vi "WRITE Config to XML file.vi"(8 "error in (no error)":errorcluster, 10 "Path":path) -> (0 "error out":errorcluster)   [LabVIEW 2015, in "Tool Module.lvlib"]
uses:
  Tool Module.lvlib
  <vilib>/Utility/xml.llb/Write to XML File(array).vi
  Tool Config/Tool Cfg.lvlib
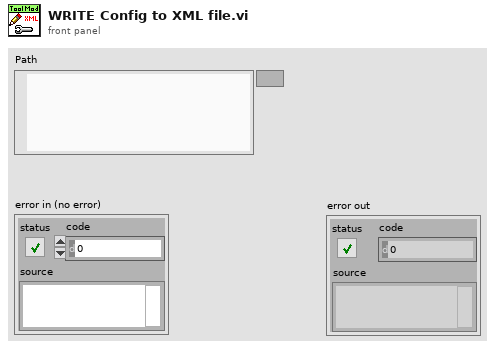
[diagram p1: front panel]
types:
  T1 = typedef "Tool Cfg.lvlib/_Configuration Cluster_v3--typedef.ctl" = cluster{"Tool Type":u16, "Tool SN":u16, "Tool Block":T2, "Motor Block":T3, "Verification Block":T4, "Probe Block":cluster{"nProbes":u16, "Probe Param Array":T5[]}}
  T2 = typedef "Tool Cfg.lvlib/_Tool Block Cluster_v3--typedef.ctl" = cluster{"Encoder Size":u16, "Encoder Scale":u32, "Encoder Offset":i32, "MaxEncoder":i32, "MinEncoder":i32, "Start Delay":sgl, "Tool Face Ref":sgl}
  T3 = typedef "Tool Cfg.lvlib/_Motor Block Cluster_v2--typedef.ctl" = cluster{"MinMotor Speed":u16, "MaxMotor Speed":u16, "Homing Speed":u16, "Jog Speed":u16, "Inspect Speed":u16, "VBlk Speed":u16, "CleaningPos":i32, "Safe Zone":i32, "Has Motor":bool, "Use Home Index":bool}
  T4 = typedef "Tool Cfg.lvlib/_Verification Blk Cluster--typedef.ctl" = cluster{"Angle":sgl, "FlankLength1":sgl, "FlankLength2":sgl, "Location":sgl, "Serial Number":u16}
  T5 = typedef "Tool Cfg.lvlib/_ProbeConfigParams Cluster--typedef.ctl" = cluster{"Name":string, "Laser Init Pwr":u16, "Laser Gain":u8, "Integ Count":u16, "Meas. Range":sgl, "Angle":sgl, "Probe Offset":sgl, "Sensor Block":T6}
  T6 = typedef "Tool Cfg.lvlib/_Sensor Block Cluster--typedef.ctl" = cluster{"nSensors":u16, "SensorCfgParams Array":T7[]}
  T7 = typedef "Tool Cfg.lvlib/_SensorConfigParams Cluster--typedef.ctl" = cluster{"Total Pixels":u16, "Positive  Peaks":bool, "CalibrCoefArray":dbl[], "Start Idx":u16, "End Idx":u16}
  T8 = typedef "Tool Cfg.lvlib/_Tool Operation Config Cluster--typedef.ctl" = cluster{"Use Tool Cfg":bool, "Use Tool Cal":bool, "Fake Data?":bool, "Mode":i16, "Array Subset Length":i16, "nArrays to Read":i16, "Full Array Read Length":i16, "nSubarrays/Sensor":i16}
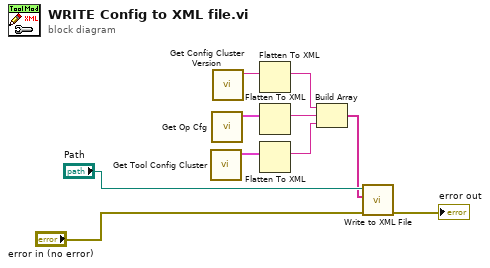
[diagram p0: block diagram]
diagram:
  n1 = call "Get Tool Config Cluster.vi"() -> ("Tool Config Cluster"=w7:T1)  [unwired: 11 in]
  n2 = call "Get Op Cfg.vi"() -> ("Tool Operation Config"=w8:T8)  [unwired: 11 in]
  n3 = call "Get Config Cluster Version.vi"() -> ("Config Cluster Version"=w1:string)  [unwired: 11 in]
  n4 = Flatten To XML(anything=w1) -> (xml string=w3:string)
  n5 = Flatten To XML(anything=w8) -> (xml string=w6:string)
  n6 = Flatten To XML(anything=w7) -> (xml string=w5:string)
  n7 = Build Array(w3, w6, w5) -> (w4:string[])
  n8 = call-poly <vilib>:"Write to XML File.vi"("error in (no error)"="error in (no error)", "XML Input"=w4, "XML File Path"="Path") -> ("error out"=→"error out":errorcluster)  [unwired: 6 in, 2 out]
